vi "fdm.vi"() -> ()   [LabVIEW 2023]
uses:
  <vilib>/express/express analysis/Spectral/Block/exnSpectralBlock spectral measurements RMS poly.vi
  <vilib>/express/express analysis/Spectral/Block/exnSpectralBlock spectral measurements RMS DDT.vi
  <vilib>/express/express analysis/Spectral/XNode/ExpressSpectralMeasurementsBlockNode.xnode
panel:
  in  "stop":bool
  out "Waveform Graph 2":dynamicdata(graph)
  out "Waveform Graph":dynamicdata(graph)
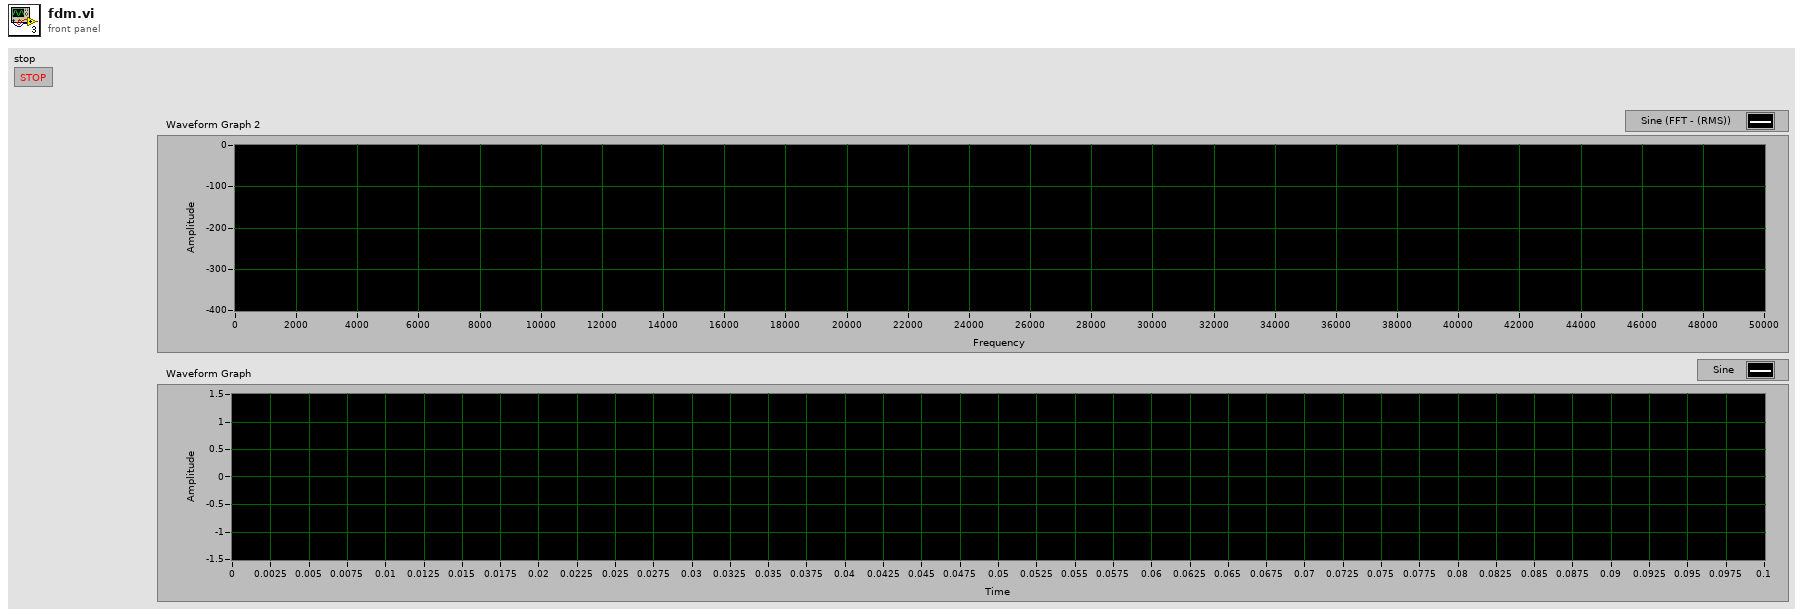
[diagram p1: front panel]
types:
  T1 = cluster{"averaging mode":u16, "weighting mode":u16, "number of averages":u32}
  T2 = cluster{"dB On (F)":bool, "unwrap phase (F)":bool, "convert to degree (F)":bool}
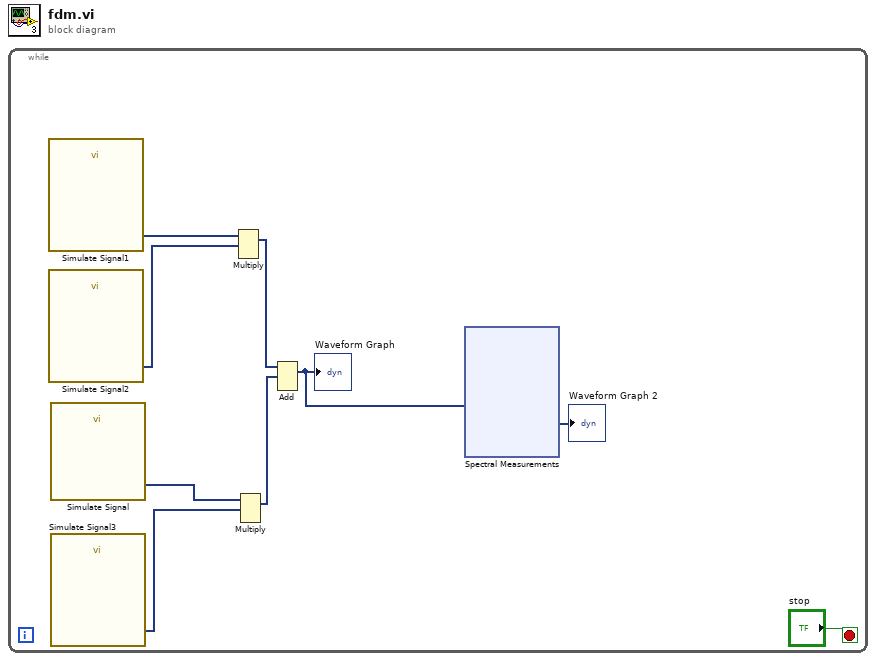
[diagram p0: block diagram]
diagram:
  n1 = while {
    stop <- "stop" stop-if-true
    n2 = call "Simulate Signal1"() -> ("Sine"=w9:dynamicdata)  [unwired: 14 in, 1 out]
    n3 = call "Simulate Signal2"() -> ("Sine"=w8:dynamicdata)  [unwired: 14 in, 1 out]
    n4 = call "Simulate Signal"() -> ("Sine"=w7:dynamicdata)  [unwired: 14 in, 1 out]
    n5 = call "Simulate Signal3"() -> ("Sine"=w6:dynamicdata)  [unwired: 14 in, 1 out]
    n6 = Multiply(1:w8, 2:w9) -> (0:w5:dynamicdata)  [unwired: 1 in, 1 out]
    n7 = Multiply(1:w6, 2:w7) -> (0:w4:dynamicdata)  [unwired: 1 in, 1 out]
    n8 = Add(1:w4, 2:w5) -> (0:w3:dynamicdata)  [unwired: 1 in, 1 out]
    "Waveform Graph" <- w3
    n9 = xnode "Spectral Measurements"("Signals"=w3) -> ("FFT - (RMS)"=→"Waveform Graph 2":dynamicdata)  [unwired: 1 in, 2 out]
  }
